vi "scale-tone-sorter.vi"(11 "Cluster":T1) -> (3 "Array":bool[][][](array[boolean]))   [LabVIEW 2019]
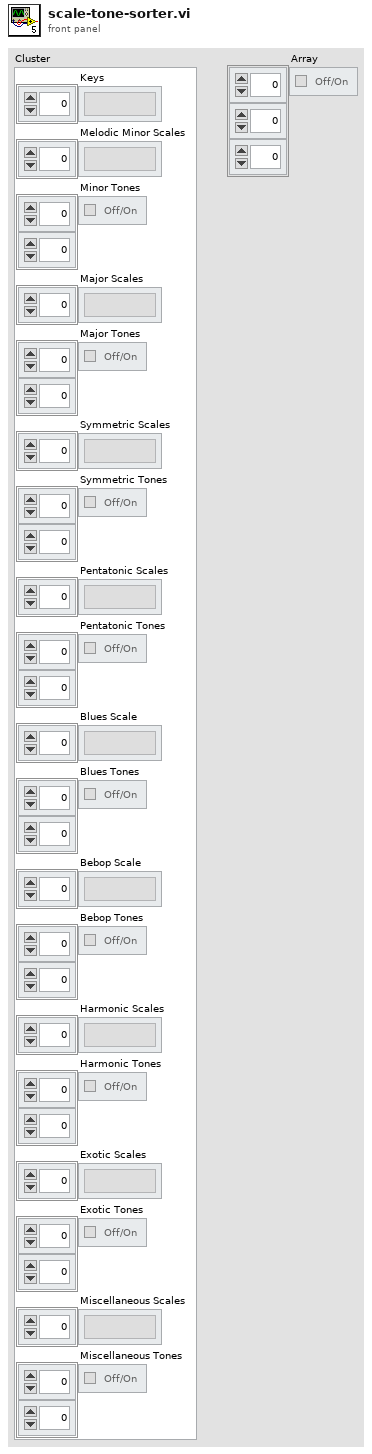
[diagram p1: front panel]
types:
  T1 = cluster{"Keys":string[], "Melodic Minor Scales":string[], "Minor Tones":bool[][], "Major Scales":string[], "Major Tones":bool[][], "Symmetric Scales":string[], "Symmetric Tones":bool[][], "Pentatonic Scales":string[], "Pentatonic Tones":bool[][], "Blues Scale":string[], "Blues Tones":bool[][], "Bebop Scale":string[], "Bebop Tones":bool[][], "Harmonic Scales":string[], "Harmonic Tones":bool[][], "Exotic Scales":string[], "Exotic Tones":bool[][], "Miscellaneous Scales":string[], "Miscellaneous Tones":bool[][]}
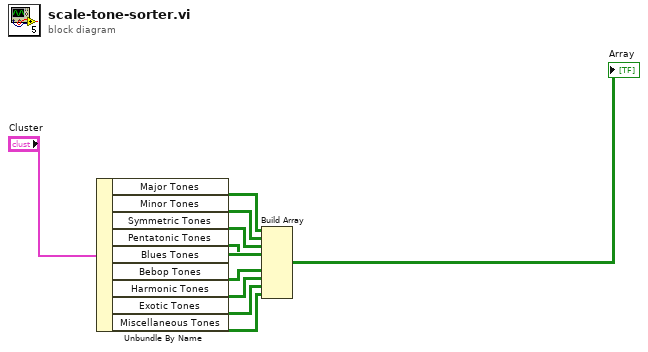
[diagram p0: block diagram]
diagram:
  n1 = Unbundle By Name("Cluster") -> ("Major Tones"=w1:bool[][], "Minor Tones"=w2:bool[][], "Symmetric Tones"=w3:bool[][], "Pentatonic Tones"=w4:bool[][], "Blues Tones"=w5:bool[][], "Bebop Tones"=w6:bool[][], "Harmonic Tones"=w7:bool[][], "Exotic Tones"=w8:bool[][], "Miscellaneous Tones"=w9:bool[][])
  n2 = Build Array(w1, w2, w3, w4, w5, w6, w7, w8, w9) -> (→"Array":bool[][][])
